vi "drawball1.vi"(4 "new picture in":picture, 6 "bdist":dbl, 7 "bflag":dbl, 9 "Y":dbl, 10 "X":dbl, 11 "bearing":dbl) -> (3 "new picture":picture)   [LabVIEW 2016]
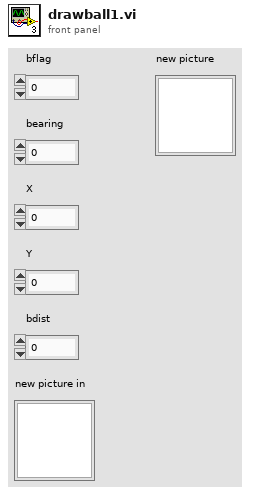
[diagram p1: front panel]
types:
  T1 = cluster{"Width":u16, "Style":enum32{"Solid", "Dash", "Dot", "DashDot", "DashDotDot"}}
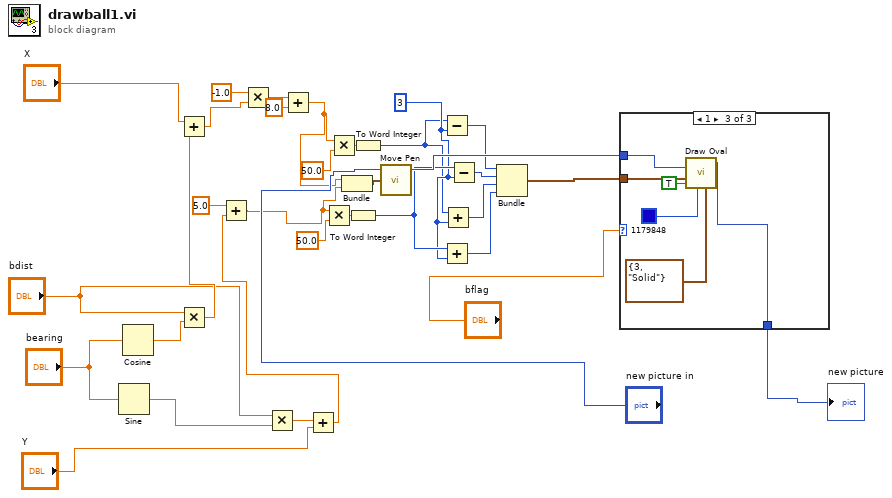
[diagram p0: block diagram]
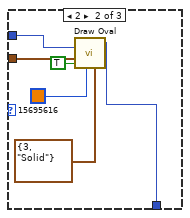
[diagram p3: hidden frame]
diagram:
  w17 = i16 3 ("Waypoint \nSize")
  n1 = Sine(x="bearing") -> (sin(x)=w3:dbl)
  n2 = Cosine(x="bearing") -> (cos(x)=w2:dbl)
  n3 = Multiply(x="bdist", y=w2) -> (x*y=w33:dbl)
  n4 = Add(x="X", y=w33) -> (x+y=w31:dbl)
  n5 = Multiply(x=-1.0, y=w31) -> (x*y=w9:dbl)
  n6 = Multiply(x="bdist", y=w3) -> (x*y=w28:dbl)
  n7 = Add(x=w9, y=8.0) -> (x+y=w6:dbl)
  n8 = Add(x=w28, y="Y") -> (x+y=w29:dbl)
  n9 = Add(x=5.0, y=w29) -> (x+y=w5:dbl)
  n10 = Multiply(x=w5, y=50.0) -> (x*y=w18:dbl)
  n11 = Multiply(x=w6, y=50.0) -> (x*y=w15:dbl)
  n12 = Bundle(w6, w5) -> (w22:cluster{dbl, dbl})  [unwired: 1 in]
  n13 = To Word Integer(number=w18) -> (16bit integer=w20:i16)
  n14 = To Word Integer(number=w15) -> (16bit integer=w16:i16)
  n15 = call <vilib>:"Move Pen.vi"("new position"=w22, "picture"="new picture in") -> ("new picture"=w23:picture)  [unwired: 3 in]
  n16 = Subtract(x=w16, y=w17) -> (x-y=w10:i16)
  n17 = Add(x=w20, y=w17) -> (x+y=w13:i16)
  n18 = Add(x=w16, y=w17) -> (x+y=w12:i16)
  n19 = Subtract(x=w20, y=w17) -> (x-y=w11:i16)
  n20 = Bundle(w10, w11, w12, w13) -> (w21:cluster{i16, i16, i16, i16})  [unwired: 1 in]
  n21 = case shown="1" "bflag" {
    tunnel: [w34 w40 w46] -> w1
    tunnel: w23 -> [w34 w38 w44]
    tunnel: w21 -> [_ w37 w43]
    frame 0, Default {
    }
    frame 2 {
      n22 = call <vilib>:"Draw Oval.vi"("picture"=w38, "rect"=w37, "fill?(F)"=TRUE, "color(black)"=u32 15695616, "pen"=T1 {"Width"=3, "Style"=enum."Solid"}) -> ("new picture"=w40:picture)  [unwired: 4 in]
    }
    frame 1 {
      n23 = call <vilib>:"Draw Oval.vi"("picture"=w44, "rect"=w43, "fill?(F)"=TRUE, "color(black)"=u32 1179848, "pen"=T1 {"Width"=3, "Style"=enum."Solid"}) -> ("new picture"=w46:picture)  [unwired: 4 in]
    }
  }
  "new picture" <- w1
